vi "Create Terminal Panel.vi"   [LabVIEW 2020]
uses:
  <vilib>/IlluminatedG/IG OOPanel/OOPanel/Manager/Manager.lvclass
  Terminal/Terminal.lvclass
  C:/Program Files (x86)/National Instruments/LabVIEW 2020/vi.lib/IlluminatedG/IG OOPanel/OOPanel/Panel/Panel.lvclass
  C:/dev/IlluminatedG/lv-stream-terminal/Terminal/Terminal/Terminal.lvclass
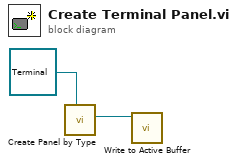
[diagram p0: block diagram]
diagram:
  n1 = call <vilib>:"Create Panel by Type.vi"("Panel Type"=refnum<class "Terminal.lvclass"> refnum ("Terminal.lvlib:Terminal.lvclass")) -> ("Panel"=w1:refnum<class "Terminal.lvclass">)  [unwired: 8 in, 2 out]
  n2 = call "Write to Active Buffer.vi"("Terminal in"=w1) -> ()  [unwired: 9 in, 2 out]
